vi "Missing Tube Count.vi"(9 "ResetMT?":bool, 10 "Max Successive":u32, 11 "Part Count in":T1) -> (3 "Boolean":bool, 5 "ArrayMissing":bool[](array[boolean]))   [LabVIEW 2021]
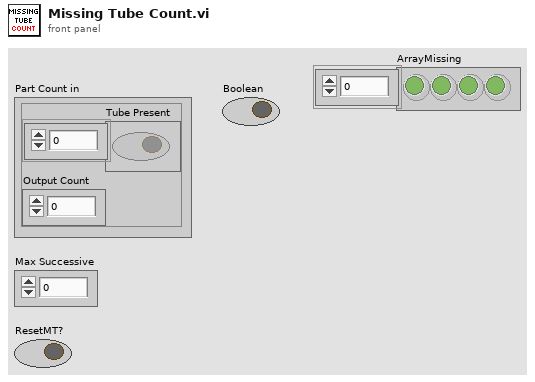
[diagram p1: front panel]
types:
  T1 = cluster{"Tube Present":bool[], "Output Count":u32}
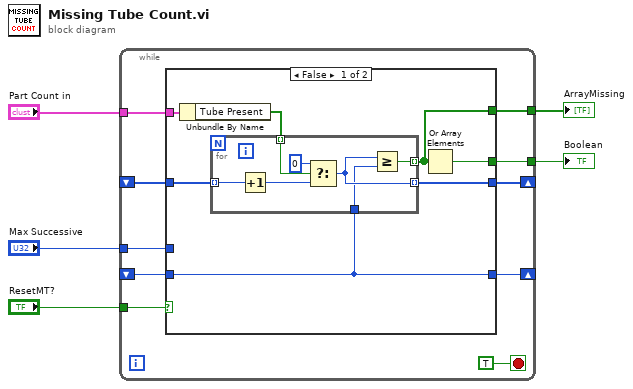
[diagram p0: block diagram]
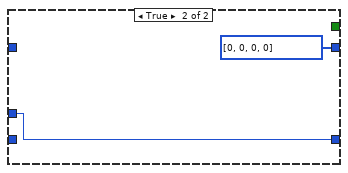
[diagram p2: hidden frame]
diagram:
  n1 = while {
    tunnel: "Part Count in" -> [w15]
    shift-right: [w13] -> _
    shift-left: _ -> [w14]
    tunnel: "Max Successive" -> [w12]
    shift-right: [w11] -> _
    shift-left: _ -> [w10]
    tunnel: [w8] -> w4
    tunnel: "ResetMT?" -> [w7]
    tunnel: [w6] -> w1
    stop <- TRUE stop-if-true
    n2 = case shown="False" w7 {
      tunnel: w15 -> [w22 _]
      tunnel: w14 -> [w21 _]
      tunnel: [w19 u32[] [0, 0, 0, 0]] -> w13
      tunnel: w12 -> [_ w31]
      tunnel: [w18 w31] -> w11
      tunnel: w10 -> [w18 _]
      tunnel: [w17 _] -> w8
      tunnel: [w16 _] -> w6
      frame False {
        n3 = Unbundle By Name(w22) -> ("Tube Present"=w20:bool[])
        n4 = for {
          tunnel: w21 -> [w28] mode=indexing
          tunnel: w20 -> [w29] mode=indexing
          tunnel: [w25] -> w19 mode=indexing
          tunnel: [w24] -> w16 mode=indexing
          tunnel: w18 -> [w23]
          n5 = Increment(x=w28) -> (x+1=w27:u32)
          n6 = Select(t=u32 0, s=w29, f=w27) -> (s? t:f=w25:u32)
          n7 = Greater Or Equal?(x=w25, y=w23) -> (x >= y?=w24:bool)
        }
        n8 = Or Array Elements(Boolean array=w16) -> (logical OR=w17:bool)
      }
      frame True {
      }
    }
  }
  "Boolean" <- w4
  "ArrayMissing" <- w1
